vi "kvCanExample1.vi"() -> ()   [LabVIEW 2022 SP3]
doc: "This VI is a very simplistic example of how to use the KVaser CAN VIs. It uses all the required VIs to initialize the KVaser CAN library, open a CAN channel and configure the channel for use. The configuration of the channel is triggered by the user pressing the \"Go Bus On\" button. \n\nAt this point two different tasks are started. The first is task transmits the specified message when the \"Send Message\" button is pressed. The second task displays the last ten messages read on the channel. It is important to note that the messages transmitted by this channel will not show up in the received list.\n\nTo reconfigure the channel, \"Go Bus Off\", change the settings, and then \"Go Bus On\".\n\nTo stop execution, press \"Go Bus Off\". When the Bus Status LED is no longer lit, press the \"STOP\" button on the panel. This ensures that the hardware interface is freed correctly for the next application to use."
panel:
  in  "error in (no error)":errorcluster
  in  "Data Bytes":u8[][](array[numeric])
  in  "Data Phase Bit Rate":i32(ring) items=["Classic 1M", "Classic 500K", "Classic 250K", "Classic 125K", "Classic 100K", "Classic 62K", "Classic 50K", "Classic 83K", "FD 500K", "FD 1M", "FD 2M", "FD 4M", "FD 8M"]
  in  "Arbitration Bit Rate":i32(ring) items=["Classic 1M", "Classic 500K", "Classic 250K", "Classic 125K", "Classic 100K", "Classic 62K", "Classic 50K", "Classic 83K", "FD 500K", "FD 1M", "FD 2M", "FD 4M", "FD 8M"]
  in  "Single Shot":bool
  in  "Bit Rate Switch":bool
  in  "FD Frame":bool
  in  "CAN FD NONISO":bool
  in  "CAN FD":bool
  in  "Accept Large DLC":bool
  in  "Wakeup":bool
  out "Read Error":errorcluster
  out "String":string
  in  "stop":bool caption="Press To End Run"
  in  "Send Message Trigger":bool
  in  "Error Frame":bool
  in  "Extended Id":bool
  in  "Standard Id":bool
  in  "Remote Frame":bool
  out "Write Error":errorcluster
  in  "DLC":u8 max=64
  in  "Message Id":u32 max=536870911 format="%.0x"
  out "error out":errorcluster
  out "Bus Status":bool
  in  "Desired Bus State":bool
  in  "Channel #":bool caption="0"
  in  "Virtual":bool
  in  "Extended":bool
  in  "Exclusive":bool
  # "Configure"
  # "Send Message"
  # "Received Messages"
  # "Time Stamp   Message Id  Flags  DLC     Data"
  # "8"
  # "16"
  # "24"
  # "32"
  # "40"
  # "48"
  # "56"
  # "64"
  # "** Do Not End Run Before Off Bus **"
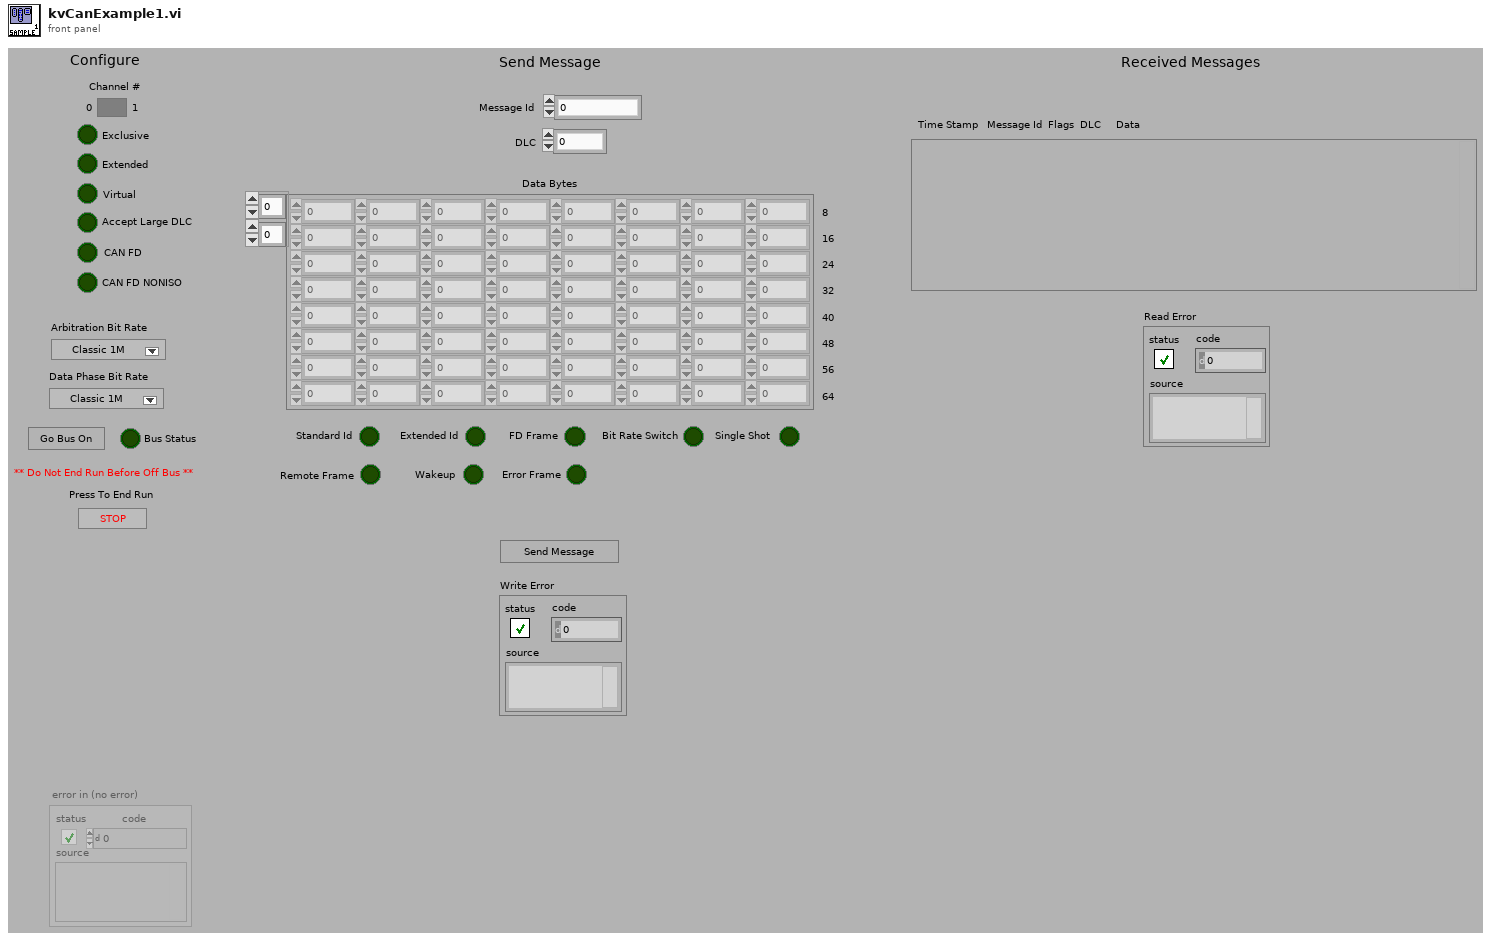
[diagram p1: front panel]
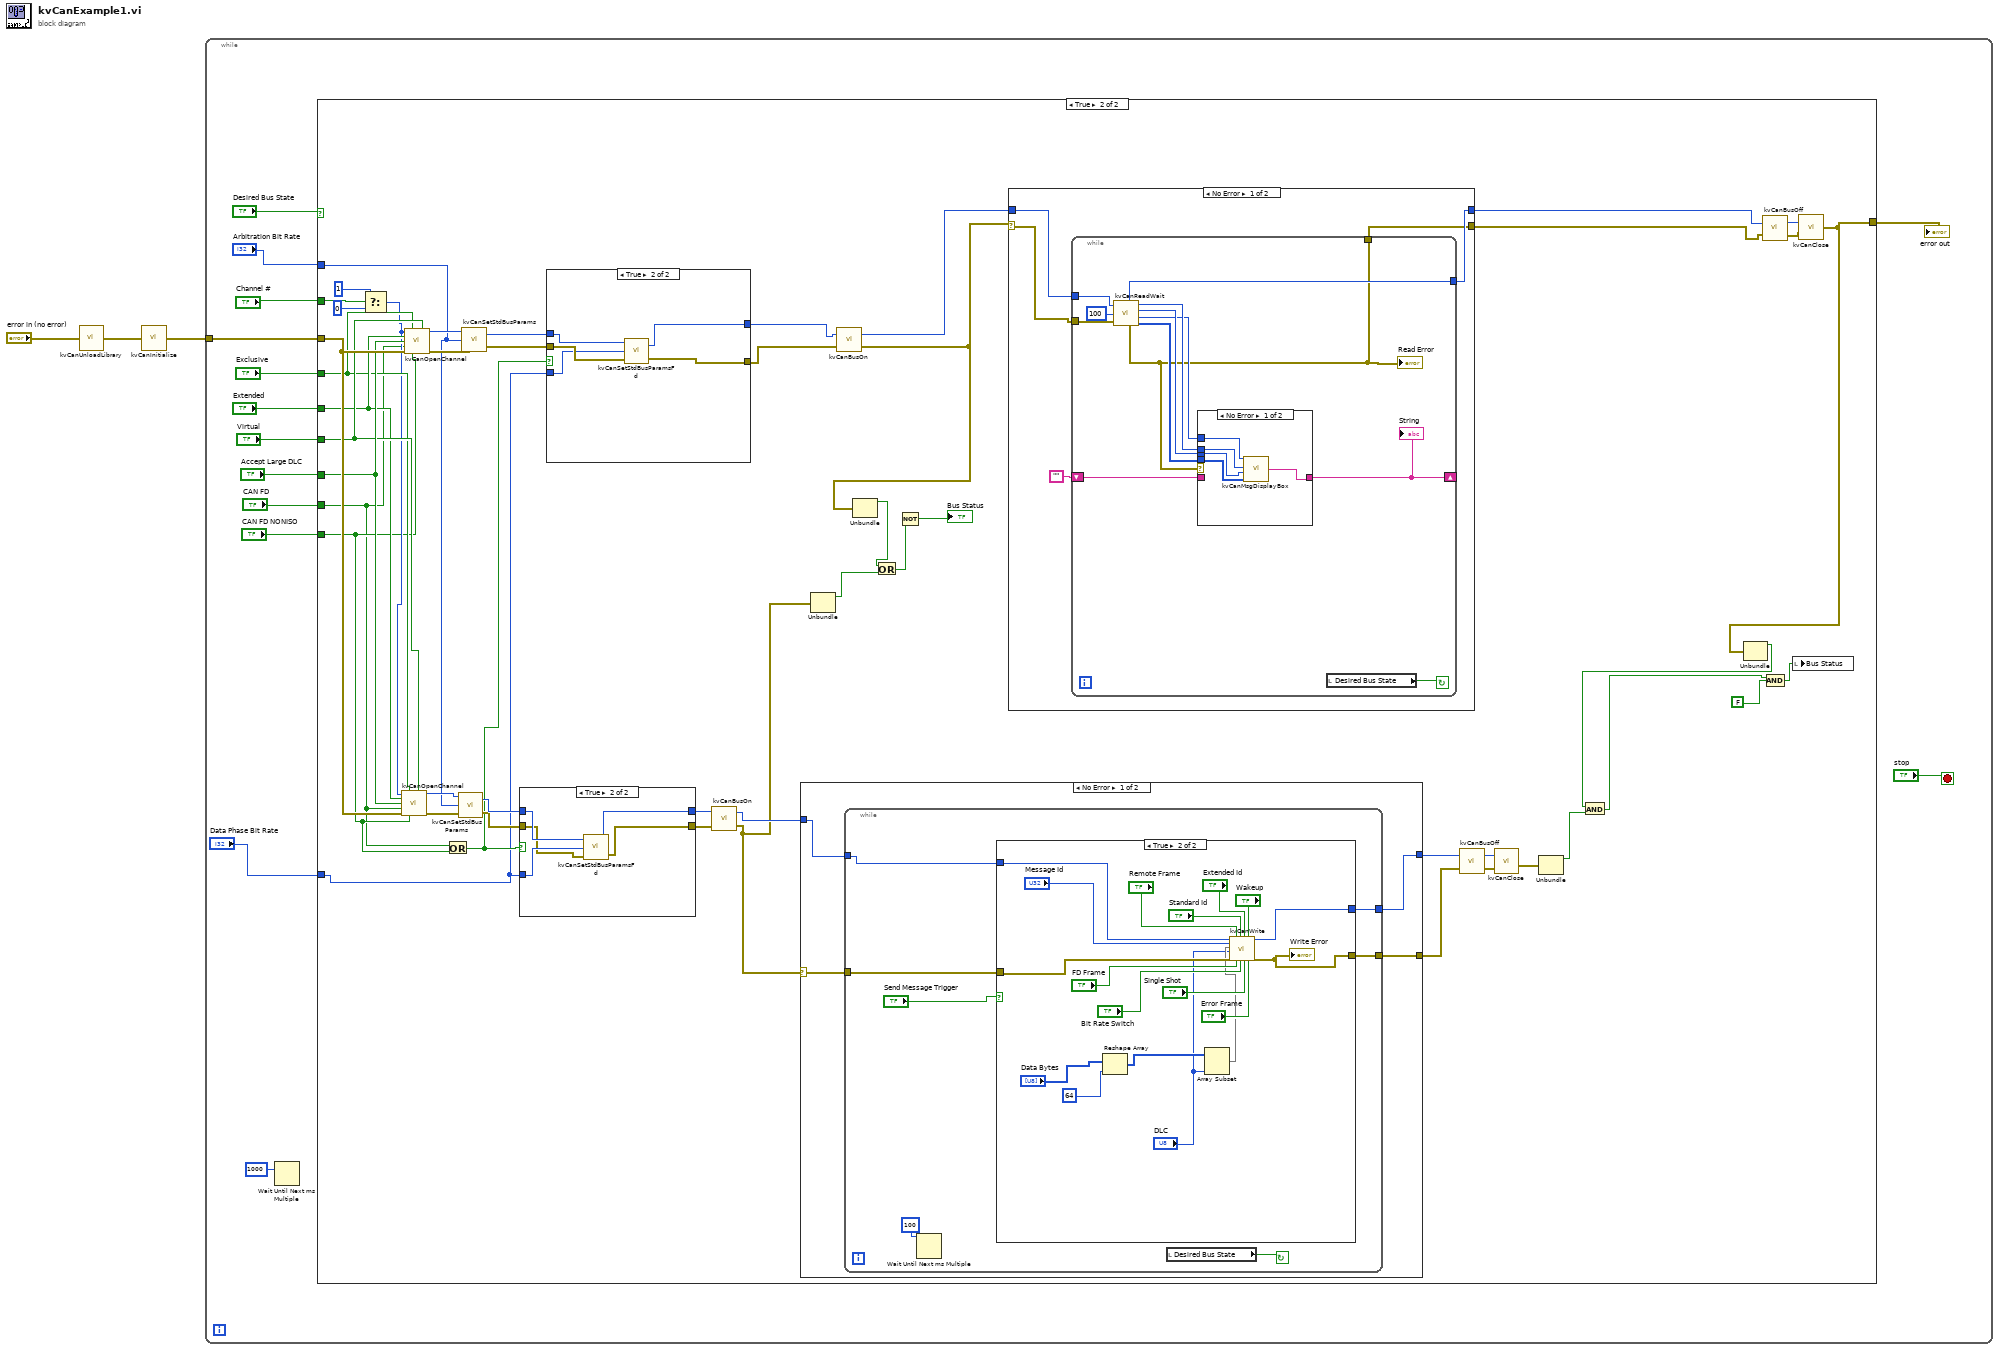
[diagram p0: block diagram]
diagram:
  n1 = call "kvCanUnloadLibrary.vi"("error in (no error)"="error in (no error)") -> ("error out"=w2:errorcluster)
  n2 = call "kvCanInitialize.vi"("error in (no error)"=w2) -> ("error out (no error)"=w3:errorcluster)
  n3 = while {
    tunnel: w3 -> [w17]
    stop <- "stop" stop-if-true
    n4 = Wait Until Next ms Multiple(millisecond multiple=u32 1000) -> ()  [unwired: 1 out]
    n5 = case shown="True" "Desired Bus State" {
      tunnel: w17 -> [w18 w49]
      tunnel: "Arbitration Bit Rate" -> [_ w50]
      tunnel: [w18 w65] -> w16
      tunnel: "Channel #" -> [_ w53]
      tunnel: "Accept Large DLC" -> [_ w48]
      tunnel: "Extended" -> [_ w46]
      tunnel: "Virtual" -> [_ w47]
      tunnel: "Exclusive" -> [_ w45]
      tunnel: "CAN FD" -> [_ w42]
      tunnel: "CAN FD NONISO" -> [_ w43]
      tunnel: "Data Phase Bit Rate" -> [_ w19]
      frame False {
      }
      frame True {
        n6 = Select(t=u32 1, s=w53, f=u32 0) -> (s? t:f=w44:u32)
        n7 = call "kvCanOpenChannel.vi"("CAN Channel Number"=w44, "WantExclusive"=w45, "AcceptVirtual"=w47, "WantExtended"=w46, "Accept Large DLC"=w48, "CAN FD"=w42, "error in (no error)"=w49, "CAN FD NONISO"=w43) -> ("Opened Channel Handle\n(output only)"=w51:i32, "error out"=w52:errorcluster)  [unwired: 6 in]
        n8 = call "kvCanOpenChannel.vi"("CAN Channel Number"=w44, "WantExclusive"=w45, "AcceptVirtual"=w47, "WantExtended"=w46, "Accept Large DLC"=w48, "CAN FD"=w42, "error in (no error)"=w49, "CAN FD NONISO"=w43) -> ("Opened Channel Handle\n(output only)"=w55:i32, "error out"=w54:errorcluster)  [unwired: 6 in]
        n9 = Or(x=w42, y=w43) -> (x .or. y?=w24:bool)
        n10 = call "kvCanSetStdBusParams.vi"("error in (no error)"=w52, "Standard CAN Baud Rate"=w50, "Channel Handle (input only)"=w51) -> ("error out"=w40:errorcluster, "Channel Handle (ouput only)"=w41:i32)
        n11 = call "kvCanSetStdBusParams.vi"("error in (no error)"=w54, "Standard CAN Baud Rate"=w50, "Channel Handle (input only)"=w55) -> ("error out"=w25:errorcluster, "Channel Handle (ouput only)"=w28:i32)
        n12 = case shown="True" w24 {
          tunnel: w41 -> [w109 w114]
          tunnel: w40 -> [w108 w112]
          tunnel: [w109 w110] -> w38
          tunnel: [w108 w111] -> w39
          tunnel: w19 -> [_ w113]
          frame False {
          }
          frame True {
            n13 = call "kvCanSetStdBusParamsFd.vi"("error in (no error)"=w112, "Standard CAN Baud Rate"=w113, "Channel Handle (input only)"=w114) -> ("error out"=w111:errorcluster, "Channel Handle (output only)"=w110:i32)
          }
        }
        n14 = case shown="True" w24 {
          tunnel: w28 -> [w69 w74]
          tunnel: [w69 w73] -> w27
          tunnel: [w68 w72] -> w26
          tunnel: w25 -> [w68 w71]
          tunnel: w19 -> [_ w70]
          frame False {
          }
          frame True {
            n15 = call "kvCanSetStdBusParamsFd.vi"("error in (no error)"=w71, "Standard CAN Baud Rate"=w70, "Channel Handle (input only)"=w74) -> ("error out"=w72:errorcluster, "Channel Handle (output only)"=w73:i32)
          }
        }
        n16 = call "kvCanBusOn.vi"("error in (no error)"=w39, "Channel Handle (input only)"=w38) -> ("error out"=w23:errorcluster, "Channel Handle (ouput only)"=w37:i32)
        n17 = case shown="No Error" w23 {
          selector: w23 -> [w75 w107]
          tunnel: [w78 w107] -> w35
          tunnel: w37 -> [w77 w106]
          tunnel: [w76 w106] -> w36
          frame No Error {
            n18 = while {
              tunnel: [w82] -> w78
              tunnel: w77 -> [w81]
              tunnel: [w80] -> w76
              tunnel: w75 -> [w79]
              stop <- w83 continue-if-true
              n19 = Wait Until Next ms Multiple(millisecond multiple=u32 100) -> ()  [unwired: 1 out]
              n20 = case shown="True" "Send Message Trigger" {
                tunnel: [w87 w105] -> w82
                tunnel: w81 -> [w86 w104]
                tunnel: [w86 w103] -> w80
                tunnel: w79 -> [w87 w102]
                frame False {
                }
                frame True {
                  n21 = Reshape Array("Data Bytes", 64 ("dimension size")) -> (w89:u8[])
                  n22 = Array Subset(array=w89, length="DLC") -> (w90:u8[])  [unwired: 1 in]
                  n23 = call "kvCanWrite.vi"("Channel Handle (input only)"=w104, "Message Id"="Message Id", "Message"=w90, "DLC"="DLC", "error in (no error)"=w102, "Remote Request"="Remote Frame", "FD Frame"="FD Frame", "Standard 11-bit Id"="Standard Id", "Bit Rate Switch"="Bit Rate Switch", "Extended 29-bit Id"="Extended Id", "Single Shot"="Single Shot", "Wakeup"="Wakeup", "Error Frame"="Error Frame") -> ("Channel Handle (output only)"=w103:i32, "error out"=w105:errorcluster)  [unwired: 5 in]
                  "Write Error" <- w105
                }
              }
              n24 = local read "Desired Bus State"() -> (w83:bool)
            }
          }
          frame Error {
          }
        }
        n25 = Unbundle(w23) -> ("status"=w22:bool)  [unwired: 2 out]
        n26 = call "kvCanBusOn.vi"("error in (no error)"=w26, "Channel Handle (input only)"=w27) -> ("error out"=w61:errorcluster, "Channel Handle (ouput only)"=w60:i32)
        n27 = Unbundle(w61) -> ("status"=w21:bool)  [unwired: 2 out]
        n28 = Or(x=w21, y=w22) -> (x .or. y?=w20:bool)
        n29 = Not(x=w20) -> (.not. x?=→"Bus Status":bool)
        n30 = case shown="No Error" w61 {
          selector: w61 -> [w117 w139]
          tunnel: [w115 w139] -> w56
          tunnel: w60 -> [w118 w138]
          tunnel: [w116 w138] -> w57
          frame No Error {
            n31 = while {
              shift-right: [w129] -> _
              shift-left: "" -> [w130]
              tunnel: w117 -> [w124]
              tunnel: w118 -> [w122]
              tunnel: [w121] -> w116
              tunnel: [w120] -> w115
              stop <- w131 continue-if-true
              n32 = call "kvCanReadWait.vi"("error in (no error)"=w124, "Read Timeout (ms)"=u32 100, "Channel Handle (input only)"=w122) -> ("Message Data"=w128:u8[], "error out"=w120:errorcluster, "Message Timestamp"=w125:u32, "Message Flags"=w127:u32, "Channel Handle (output only)"=w121:i32, "Message Id"=w126:i32)
              "Read Error" <- w120
              n33 = case shown="No Error" w120 {
                tunnel: w130 -> [_ w137]
                tunnel: [w136 w137] -> w129
                tunnel: w128 -> [w135 _]
                tunnel: w127 -> [w134 _]
                tunnel: w126 -> [w133 _]
                tunnel: w125 -> [w132 _]
                frame No Error {
                  n34 = call "kvCanMsgDisplayBox.vi"("Message Data"=w135, "Message Flags"=w134, "Message Id"=w133, "Time Stamp"=w132) -> ("Output String"=w136:string)
                }
                frame Error {
                }
              }
              "String" <- w129
              n35 = local read "Desired Bus State"() -> (w131:bool)
            }
          }
          frame Error {
          }
        }
        n36 = call "kvCanBusOff.vi"("error in (no error)"=w35, "Channel Handle (input only)"=w36) -> ("error out"=w34:errorcluster, "Channel Handle (ouput only)"=w33:i32)
        n37 = call "kvCanClose.vi"("error in (no error)"=w34, "Channel Handle (input only)"=w33) -> ("error out"=w32:errorcluster)
        n38 = Unbundle(w32) -> ("status"=w30:bool)  [unwired: 2 out]
        n39 = call "kvCanBusOff.vi"("error in (no error)"=w56, "Channel Handle (input only)"=w57) -> ("error out"=w58:errorcluster, "Channel Handle (ouput only)"=w59:i32)
        n40 = call "kvCanClose.vi"("error in (no error)"=w58, "Channel Handle (input only)"=w59) -> ("error out"=w65:errorcluster)
        n41 = Unbundle(w65) -> ("status"=w31:bool)  [unwired: 2 out]
        n42 = And(x=w31, y=w30) -> (x .and. y?=w29:bool)
        n43 = And(x=w29, y=FALSE) -> (x .and. y?=w63:bool)
        n44 = local write "Bus Status"(w63) -> ()
      }
    }
    "error out" <- w16
  }
